vi "addressing_conversion.vi"(11 "addressing_type":T1) -> (3 "addressing_number":u32 format="%x")   [LabVIEW 2014, in "Dali_usb.lvlib"]
uses:
  Dali_usb.lvlib
  Controls/Addressing_type.ctl
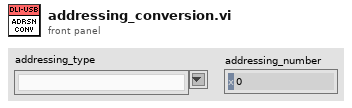
[diagram p1: front panel]
types:
  T1 = typedef "Dali_usb.lvlib/Addressing_type.ctl" = string
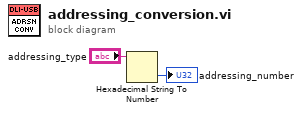
[diagram p0: block diagram]
diagram:
  n1 = Hexadecimal String To Number(string="addressing_type") -> (number=→"addressing_number":u32)  [unwired: 2 in, 1 out]
